vi "CalibrateAll.vi"() -> ()   [LabVIEW 2021]
uses:
  include/GlobalVariables.vi
  Other Models/EFD Ultimus V/EFD Ultimus V.lvlib
panel:
  in  "HBtrayComponent":enum16{"BP", "Si", "HB", "HBonBP", "Other"}(ring)=enum."HB"
  out "Status4":bool
  in  "Si/HB Calibration":bool
  out "SiHB XYZU":string
  in  "Autofocus2":T1={"Enable"=TRUE, "InitialStepSize"=0.05, "Tolerance"=0.02, "Abort"=FALSE} {"Tolerance" format="%#_13g"}
  in  "SaveImagesLog 2":bool
  in  "VisibilityInCamera2":enum16{"JoyStick", "AllVisible"}(ring)=enum."AllVisible"
  in  "SiTrayComponent":enum16{"Si", "SiOnBP"}(ring)
  in  "Operation":enum16{"Manual", "Automatic"}(ring)=enum."Automatic"
  in  "GlueAmtCalib":bool
  in  "PaperWt(g)":dbl
  in  "PaperWtWithGlue(g)":dbl
  out "AmtDispensed(g)":dbl
  in  "WtFor50Psi30Sec":dbl=1.039
  out "CorrectionFactor":dbl=1.0
  out "PressureWillBeSetTo":dbl[](array[numeric])
  in  "DefaultPressure":dbl[](array[numeric])=[30.0, 21.0, 32.0, 22.0]
  in  "Calc":bool
  out "?":bool
  in  "VISA resource name":refnum<visa-resource-name>="COM8"
  out "Status5":bool
  in  "Switches":T2
  out "VacState2":T3
  out "VacState1":T4
  out "HighVSPosition":picture
  out "Status3":bool
  out "BP XYZU":string
  in  "SaveImagesLog":bool
  in  "Autofocus":T1={"Enable"=TRUE, "InitialStepSize"=0.05, "Tolerance"=0.02, "Abort"=FALSE} {"Tolerance" format="%#_13g"}
  in  "VisibilityInCamera":enum16{"JoyStick", "AllVisible"}(ring)=enum."AllVisible"
  in  "Component":T5(ring)=enum."BP_CuEdges"
  in  "BP_calibration":bool
  in  "Operation":enum16{"Manual", "Automatic"}(ring)=enum."Automatic"
  out "Status2":bool
  in  "SyringeToPlateGap(mm)":dbl=0.35
  out "FinalZ":dbl
  in  "PD_Z":bool=TRUE
  in  "AutoFocus":bool=TRUE
  in  "SyringeZCalibration":bool
  out "Status1":bool
  in  "ControlType":T6(ring)
  in  "VacuumControl":bool
  in  "StopImageDisplay":bool
  out "error out":errorcluster
  out "Image 2":T7[](array[plugin-control]) caption="BP_calibration"
  out "Image":T7(plugin-control)
  in  "ModuleName":string="T1"
  in  "AssmbType":enum16{"Sensor", "HB"}(ring)
  in  "Error In":errorcluster
  in  "Position":enum16{"1", "2"}(ring)
  in  "Zone":enum16{"ZoneA", "ZoneB", "ZoneC", "ZoneD"}(ring)
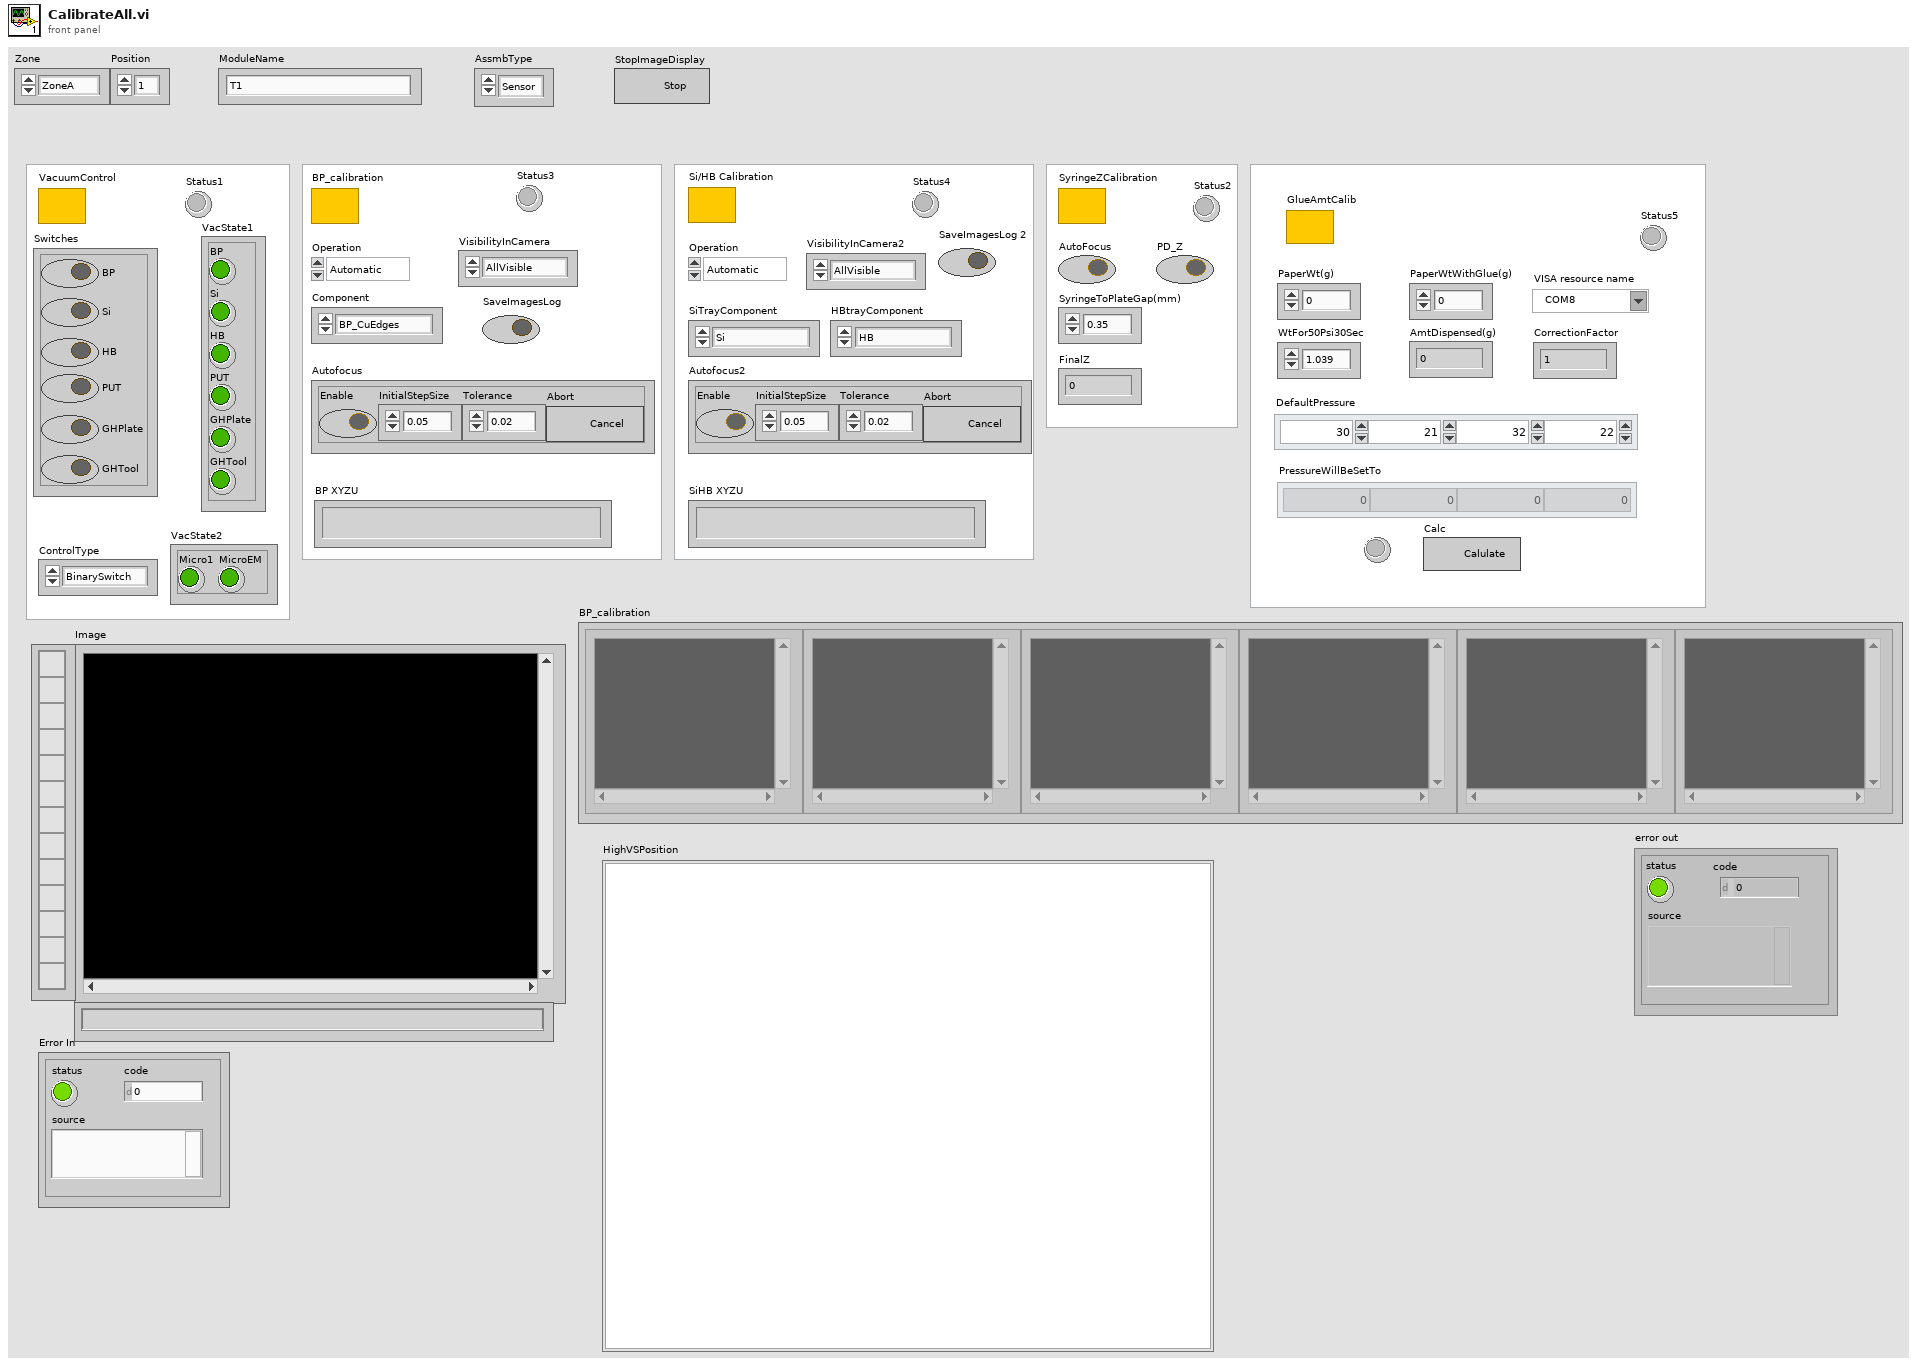
[diagram p1: front panel]
types:
  T1 = cluster{"Enable":bool, "InitialStepSize":dbl, "Tolerance":dbl, "Abort":bool}
  T2 = cluster{"BP":bool, "Si":bool, "HB":bool, "PUT":bool, "GHPlate":bool, "GHTool":bool}
  T3 = cluster{"Micro1":bool, "MicroEM":bool, "data[2]":bool, "data[3]":bool, "data[4]":bool, "data[5]":bool, "data[6]":bool, "data[7]":bool, "data[8]":bool}
  T4 = cluster{"BP":bool, "Si":bool, "HB":bool, "PUT":bool, "GHPlate":bool, "GHTool":bool, "data[6]":bool, "data[7]":bool, "data[8]":bool}
  T5 = enum16{"BP_BackLight", "Si", "SiOnBP", "HB", "HBOnBPSi", "BP_CuEdges", "Other"}
  T6 = enum16{"BinarySwitch", "DecimalSwitch", "Conversion"}
  T7 = typedef "IMAQ Image.ctl" = refnum<image>
  T8 = cluster{"Baud Rate ":u32, "Parity ":u16, "Data Bits ":u16, "Stop Bits":u16}
  T9 = enum16{"open", "replace", "create", "open or create", "replace or create", "replace or create with confirmation"}
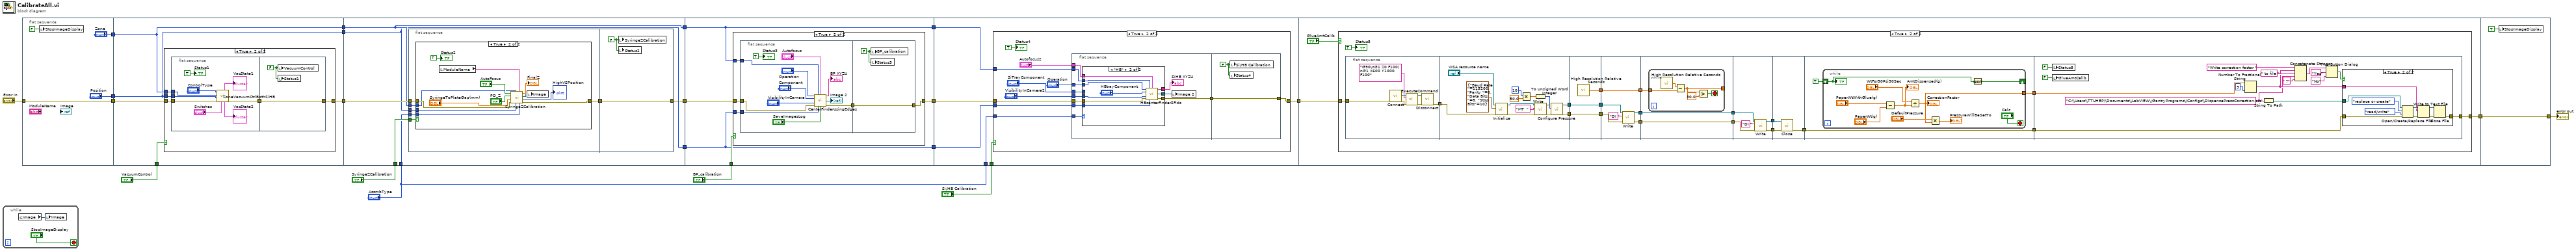
[diagram p0: block diagram]
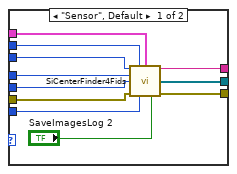
[diagram p6: hidden frame]
diagram:
  n1 = while {
    stop <- "StopImageDisplay" stop-if-true
    n2 = global read "GlobalVariables.vi" "Image"() -> (w23:T7)
    n3 = local write "Image"(w23) -> ()
  }
  n4 = flat-sequence {
    tunnel: "Error In" -> [w27]
    tunnel: ["Position"] -> w16
    tunnel: ["Zone"] -> w15
    tunnel: [w27] -> w14
    tunnel: [w32] -> w21
    tunnel: [w30] -> w18
    tunnel: [w29] -> w17
    tunnel: w16 -> [w29]
    tunnel: w15 -> [w30]
    tunnel: w14 -> [w31]
    tunnel: "VacuumControl" -> [w28]
    tunnel: w21 -> [w56]
    tunnel: "SyringeZCalibration" -> [w55]
    tunnel: w18 -> [w54]
    tunnel: w17 -> [w53]
    tunnel: [w54] -> w12
    tunnel: [w53] -> w11
    tunnel: [w52] -> w9
    tunnel: "AssmbType" -> [w50]
    tunnel: w12 -> [w80]
    tunnel: w11 -> [w79]
    tunnel: "BP_calibration" -> [w83]
    tunnel: w9 -> [w82]
    tunnel: [w81] -> w7
    tunnel: [w80] -> w6
    tunnel: [w79] -> w5
    tunnel: "AssmbType" -> [w109]
    tunnel: w7 -> [w108]
    tunnel: w6 -> [w107]
    tunnel: w5 -> [w106]
    tunnel: "Si/HB Calibration" -> [w105]
    tunnel: [w104] -> w2
    tunnel: w2 -> [w158]
    tunnel: [w156] -> w1
    tunnel: [w266] -> w3
    tunnel: w1 -> [w266]
    frame #0 {
      n5 = local write "StopImageDisplay"(FALSE ("StopImageDisplay")) -> ()
    }
    frame #1 {
      n6 = case shown="True" w28 {
        tunnel: w29 -> [_ w38]
        tunnel: w30 -> [_ w37]
        tunnel: [w33 w36] -> w32
        tunnel: w31 -> [w33 w35]
        frame False {
        }
        frame True {
          n7 = flat-sequence {
            tunnel: w38 -> [w47]
            tunnel: w37 -> [w46]
            tunnel: w35 -> [w43]
            tunnel: [w44] -> w34
            tunnel: [w49] -> w36
            tunnel: w34 -> [w49]
            frame #0 {
              n8 = call "ZoneVacuumCtrlBothSiHB.vi"("Switches"="Switches", "Error In"=w43, "Position"=w47, "Zone"=w46, "ControlType"="ControlType") -> ("Error Out"=w44:errorcluster, "VacState2"=→"VacState2":T3, "VacState1"=→"VacState1":T4)  [unwired: 2 in, 2 out]
              "Status1" <- TRUE ("Status1")
            }
            frame #1 {
              w48 = FALSE ("VacuumControl")
              n9 = local write "VacuumControl"(w48) -> ()
              n10 = local write "Status1"(w48) -> ()
            }
          }
        }
      }
    }
    frame #2 {
      n11 = flat-sequence {
        tunnel: w56 -> [w62]
        tunnel: w55 -> [w61]
        tunnel: w54 -> [w60]
        tunnel: w53 -> [w59]
        tunnel: [w58] -> w51
        tunnel: w50 -> [w57]
        tunnel: [w78] -> w52
        tunnel: w51 -> [w78]
        frame #0 {
          n12 = case shown="True" w61 {
            tunnel: w62 -> [w63 w76]
            tunnel: w60 -> [_ w73]
            tunnel: w59 -> [_ w72]
            tunnel: [w63 w68] -> w58
            tunnel: w57 -> [_ w67]
            frame False {
            }
            frame True {
              n13 = local read "ModuleName"() -> (w69:string)
              n14 = call "SyringeZCalibration.vi"("AssmbType"=w67, "ModuleName"=w69, "Position"=w72, "Zone"=w73, "Error In"=w76, "SyringeToPlateGap(mm)"="SyringeToPlateGap(mm)", "PD_Z"="PD_Z", "AutoFocus"="AutoFocus") -> ("error out"=w68:errorcluster, "HighVSPosition"=→"HighVSPosition":picture, "Image"=w70:T7, "FinalZ"=→"FinalZ":dbl)
              n15 = local write "Image"(w70) -> ()
              "Status2" <- TRUE ("Status2")
            }
          }
        }
        frame #1 {
          w77 = FALSE ("SyringeZCalibration")
          n16 = local write "SyringeZCalibration"(w77) -> ()
          n17 = local write "Status2"(w77) -> ()
        }
      }
    }
    frame #3 {
      n18 = case shown="True" w83 {
        tunnel: w80 -> [_ w89]
        tunnel: w79 -> [_ w88]
        tunnel: w82 -> [w84 w87]
        tunnel: [w84 w86] -> w81
        frame False {
        }
        frame True {
          n19 = flat-sequence {
            tunnel: w89 -> [w98]
            tunnel: w88 -> [w97]
            tunnel: w87 -> [w93]
            tunnel: [w92] -> w85
            tunnel: [w103] -> w86
            tunnel: w85 -> [w103]
            frame #0 {
              n20 = call "CenterFinderUsingEdges.vi"("Operation"="Operation", "Zone"=w98, "Autofocus"="Autofocus", "Component"="Component", "VisibilityInCamera"="VisibilityInCamera", "error in (no error)"=w93, "Position"=w97, "SaveImagesLog"="SaveImagesLog") -> ("Output XYZU"=→"BP XYZU":string, "Image 2"=→"Image 2":T7[], "error out"=w92:errorcluster)  [unwired: 4 in, 1 out]
              "Status3" <- TRUE ("Status3")
            }
            frame #1 {
              w102 = FALSE ("BP_calibration")
              n21 = local write "BP_calibration"(w102) -> ()
              n22 = local write "Status3"(w102) -> ()
            }
          }
        }
      }
    }
    frame #4 {
      n23 = case shown="True" w105 {
        tunnel: w109 -> [_ w121]
        tunnel: w108 -> [w110 w120]
        tunnel: w107 -> [_ w119]
        tunnel: w106 -> [_ w118]
        tunnel: [w110 w114] -> w104
        frame False {
        }
        frame True {
          n24 = flat-sequence {
            tunnel: w121 -> [w132]
            tunnel: w120 -> [w131]
            tunnel: w119 -> [w130]
            tunnel: w118 -> [w129]
            tunnel: "VisibilityInCamera2" -> [w128]
            tunnel: "Autofocus2" -> [w127]
            tunnel: [w124] -> w115
            tunnel: "Operation" -> [w123]
            tunnel: "SiTrayComponent" -> [w122]
            tunnel: w115 -> [w155]
            tunnel: [w155] -> w114
            frame #0 {
              n25 = case shown="\"HB\"" w132 {
                tunnel: w131 -> [w143 w152]
                tunnel: w130 -> [w142 w150]
                tunnel: w129 -> [w141 w151]
                tunnel: w128 -> [w139 w153]
                tunnel: w127 -> [w138 w149]
                tunnel: [w137 w147] -> w126
                tunnel: [w136 w148] -> w125
                tunnel: [w135 w146] -> w124
                tunnel: w123 -> [w134 w145]
                tunnel: w122 -> [w133 _]
                frame "Sensor", Default {
                  n26 = call "SiCenterFinder4Fids.vi"("Operation"=w134, "Zone"=w142, "Autofocus"=w138, "Component"=w133, "VisibilityInCamera"=w139, "error in (no error)"=w143, "Position"=w141, "SaveImagesLog"="SaveImagesLog 2") -> ("Output XYZU"=w136:string, "Image 2"=w137:T7[], "error out"=w135:errorcluster)  [unwired: 4 in, 1 out]
                }
                frame "HB" {
                  n27 = call "HBcenterFinder2Fids.vi"("Operation"=w145, "Zone"=w150, "Autofocus"=w149, "Component"="HBtrayComponent", "VisibilityInCamera"=w153, "error in (no error)"=w152, "Position"=w151) -> ("Output XYZU"=w148:string, "Image 2"=w147:T7[], "error out"=w146:errorcluster)  [unwired: 5 in, 1 out]
                }
              }
              "SiHB XYZU" <- w125
              n28 = local write "Image 2"(w126) -> ()
            }
            frame #1 {
              w154 = FALSE ("Si/HB Calibration")
              n29 = local write "Si/HB Calibration"(w154) -> ()
              n30 = local write "Status4"(w154) -> ()
            }
          }
          "Status4" <- TRUE ("Status4")
        }
      }
    }
    frame #5 {
      n31 = case shown="True" "GlueAmtCalib" {
        tunnel: w158 -> [w159 w164]
        tunnel: [w159 w161] -> w156
        frame False {
        }
        frame True {
          n32 = flat-sequence {
            tunnel: [w180] -> w178
            tunnel: w164 -> [w179]
            tunnel: [w187] -> w177
            tunnel: [w188] -> w176
            tunnel: w178 -> [w186]
            tunnel: [w202] -> w175
            tunnel: [w201] -> w174
            tunnel: [w200] -> w173
            tunnel: w177 -> [w202]
            tunnel: w176 -> [w201]
            tunnel: [w206] -> w172
            tunnel: [w205] -> w171
            tunnel: w175 -> [w208]
            tunnel: w174 -> [w207]
            tunnel: [w203] -> w170
            tunnel: w173 -> [w203]
            tunnel: w172 -> [w211]
            tunnel: w171 -> [w210]
            tunnel: [w211] -> w169
            tunnel: [w210] -> w168
            tunnel: w170 -> [w209]
            tunnel: w169 -> [w220]
            tunnel: w168 -> [w221]
            tunnel: [w219] -> w167
            tunnel: [w218] -> w166
            tunnel: w167 -> [w224]
            tunnel: w166 -> [w223]
            tunnel: [w222] -> w165
            tunnel: w165 -> [w227]
            tunnel: [w227] -> w162
            tunnel: [w225] -> w160
            tunnel: [w243] -> w161
            tunnel: w162 -> [w249]
            tunnel: w160 -> [w248]
            frame #0 {
              n33 = call "Connect.vi"("error in (no error)"=w179) -> ("error out"=w184:errorcluster, "controller"=w185:refnum<k24>)  [unwired: 9 in]
              n34 = call "ExecuteCommand.vi"("error in (no error)"=w184, "Command Code"="G90\nG1 Z0 F100\nG1 X600 Y1000 F100", "controller in"=w185) -> ("error out"=w182:errorcluster, "controller out"=w183:refnum<k24>)  [unwired: 6 in, 1 out]
              n35 = call "Disconnect.vi"("error in (no error)"=w182, "controller"=w183) -> ("error out"=w180:errorcluster)  [unwired: 9 in]
            }
            frame #1 {
              n36 = call "Initialize.vi"("error in (no error)"=w186, "Serial Configuration"=T8 {"Baud Rate "=115200, "Parity "=0, "Data Bits "=8, "Stop Bits"=10}, "VISA resource name"="VISA resource name") -> ("error out"=w194:errorcluster, "VISA resource name out"=w193:refnum<visa-resource-name>)  [unwired: 7 in]
              n37 = Multiply(x=10, y=50.0 ("PressureSet")) -> (x*y=w196:dbl)
              n38 = To Unsigned Word Integer(number=w196) -> (unsigned 16bit integer=w197:u16)
              n39 = call "Write.vi"("error in (no error)"=w194, "Command To Write"="MT  ", "VISA resource name"=w193) -> ("error out"=w198:errorcluster, "VISA resource name out"=w195:refnum<visa-resource-name>)  [unwired: 7 in]
              n40 = call "Configure Pressure.vi"("error in (no error)"=w198, "Pressure Setting (0000)"=w197, "VISA resource name"=w195) -> ("error out"=w188:errorcluster, "VISA resource name out"=w187:refnum<visa-resource-name>)  [unwired: 7 in]
            }
            frame #2 {
              n41 = call <vilib>:"High Resolution Relative Seconds.vi"() -> ("relative seconds"=w200:dbl)
            }
            frame #3 {
              n42 = call "Write.vi"("error in (no error)"=w207, "Command To Write"="DI ", "VISA resource name"=w208) -> ("error out"=w205:errorcluster, "VISA resource name out"=w206:refnum<visa-resource-name>)  [unwired: 7 in]
            }
            frame #4 {
              n43 = while {
                tunnel: w209 -> [w215]
                tunnel: [w212] -> _
                stop <- w214 stop-if-true
                n44 = call <vilib>:"High Resolution Relative Seconds.vi"() -> ("relative seconds"=w216:dbl)
                n45 = Subtract(x=w216, y=w215) -> (x-y=w212:dbl)
                n46 = Greater?(x=w212, y=30.0 ("Time(s)")) -> (0:w214:bool)
              }
            }
            frame #5 {
              n47 = call "Write.vi"("error in (no error)"=w221, "Command To Write"="DI ", "VISA resource name"=w220) -> ("error out"=w219:errorcluster, "VISA resource name out"=w218:refnum<visa-resource-name>)  [unwired: 7 in]
            }
            frame #6 {
              n48 = call "Close.vi"("error in (no error)"=w224, "VISA resource name"=w223) -> ("error out"=w222:errorcluster)  [unwired: 9 in]
            }
            frame #7 {
              n49 = while {
                shift-right: [w229] -> _
                shift-left: TRUE -> [w230]
                tunnel: [w228] -> w225
                stop <- "Calc" stop-if-true
                n50 = Subtract(x="PaperWtWithGlue(g)", y="PaperWt(g)") -> (x-y=w233:dbl)
                "AmtDispensed(g)" <- w233
                n51 = Divide(x="WtFor50Psi30Sec", y=w233) -> (x/y=w228:dbl)
                "CorrectionFactor" <- w228
                n52 = Multiply(x="DefaultPressure", y=w228) -> (x*y=→"PressureWillBeSetTo":dbl[])
                n53 = Not(x=w230) -> (.not. x?=w229:bool)
                "?" <- w230
              }
            }
            frame #8 {
              w240 = "C:\\Users\\TTUHEP\\Documents\\LabVIEW\\GantryPrograms\\Configs\\DispensePressCorrection.txt" ("string")
              n54 = local write "Status5"(FALSE ("Status5")) -> ()
              n55 = local write "GlueAmtCalib"(FALSE ("GlueAmtCalib")) -> ()
              n56 = Number To Fractional String(number=w248, precision (6)=i16 3) -> (F-format string=w241:string)  [unwired: 2 in]
              n57 = String To Path(string=w240) -> (path=w239:path)
              n58 = Concatenate Strings("Write correction factor ", w241, " to file ", w240, " ?" ("string")) -> (w244:string)
              n59 = Two Button Dialog(message=w244, 1:"No" ("Center Button Text (\"No\")"), 2:"Yes" ("Left Button Text (\"Yes\")")) -> (T button?=w242:bool)
              n60 = case shown="True" w242 {
                tunnel: w249 -> [w254 w264]
                tunnel: [w254 w257] -> w243
                tunnel: w241 -> [_ w256]
                tunnel: w239 -> [_ w255]
                frame False {
                }
                frame True {
                  n61 = Open/Create/Replace File(file path (use dialog)=w255, error in=w264, operation (0:open)=T9."replace or create", access (0:read/write)=enum16{"read/write", "read-only", "write-only"}."read/write") -> (refnum out=w260:refnum<file>, error out=w261:errorcluster)  [unwired: 2 in, 1 out]
                  n62 = Write to Text File(file (use dialog)=w260, text=w256, error in=w261) -> (refnum out=w263:refnum<file>, error out=w262:errorcluster)  [unwired: 1 in, 1 out]
                  n63 = Close File(refnum=w263, error in=w262) -> (error out=w257:errorcluster)  [unwired: 1 out]
                }
              }
            }
          }
          "Status5" <- TRUE ("Status5")
        }
      }
    }
    frame #6 {
      n64 = local write "StopImageDisplay"(TRUE ("StopImageDisplay")) -> ()
    }
  }
  "error out" <- w3
